vi "MRC Free String.vi"(8 "error in (no error)":errorcluster, 11 "mrcString":cluster{"str":u64, "len":i64}) -> (0 "error out":errorcluster)   [LabVIEW 2026, in "MrcLib.lvlib"]
doc: "void MRC_CALLCONV MRC_FreeString(const struct MRC_String* mrcString);"
uses:
  MrcLib.lvlib
  MrcLib.dll
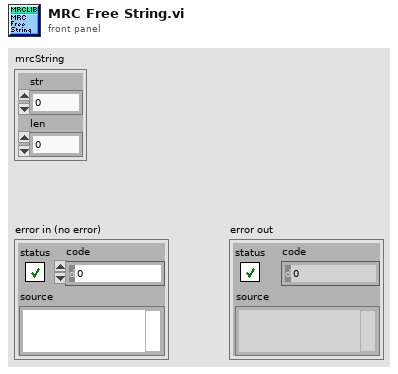
[diagram p1: front panel]
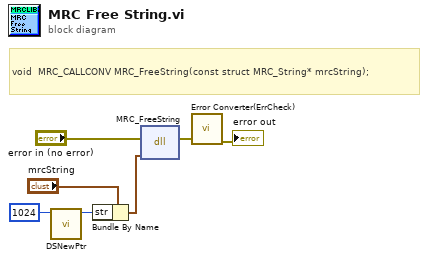
[diagram p0: block diagram]
diagram:
  # "void  MRC_CALLCONV MRC_FreeString(const struct MRC_String* mrcString);"
  n1 = call <vilib>:"DSNewPtr.vi"("Size"=u64 1024) -> ("Pointer"=w5:u64)  [unwired: 9 in, 1 out]
  n2 = Bundle By Name(cluster="mrcString", "str"=w5) -> (w4:cluster{"str":u64, "len":i64})
  n3 = dll-call lib="MrcLib.*" fn="MRC_FreeString"(error in="error in (no error)", "mrcString"=w4) -> (error out=w2:errorcluster)  [unwired: 4 in, 1 out]
  n4 = call <vilib>:"Error Converter(ErrCheck).vi"("error in (no error)"=w2) -> ("error out"=→"error out":errorcluster)  [unwired: 10 in]
